vi "test_WFGenerate01DC.vi"() -> ()   [LabVIEW 2013]
panel:
  out "Waveform Out":waveform(dbl)={"t0"=timestamp(0 s since 1904-01-01), "dt"=5e-05, "Y"=array[10000 elements]}
  in  "Param 3":dbl=1000.0
  in  "Param 2":dbl=1000.0
  in  "Param 1":dbl=1000.0
  in  "Param 0":dbl=1000.0
  in  "Waveform Properties":T1={"Fs (Hz)"=20000.0, "Amplitude (V)"=5.0, "Ramp (s)"=0.02, "Duration (s)"=0.5} {"Ramp (s)" min=0.0; "Fs (Hz)" min=0.0}
  out "Waveform Graph":waveform(dbl)(graph)={"t0"=timestamp(0 s since 1904-01-01), "dt"=5e-05, "Y"=array[10000 elements]}
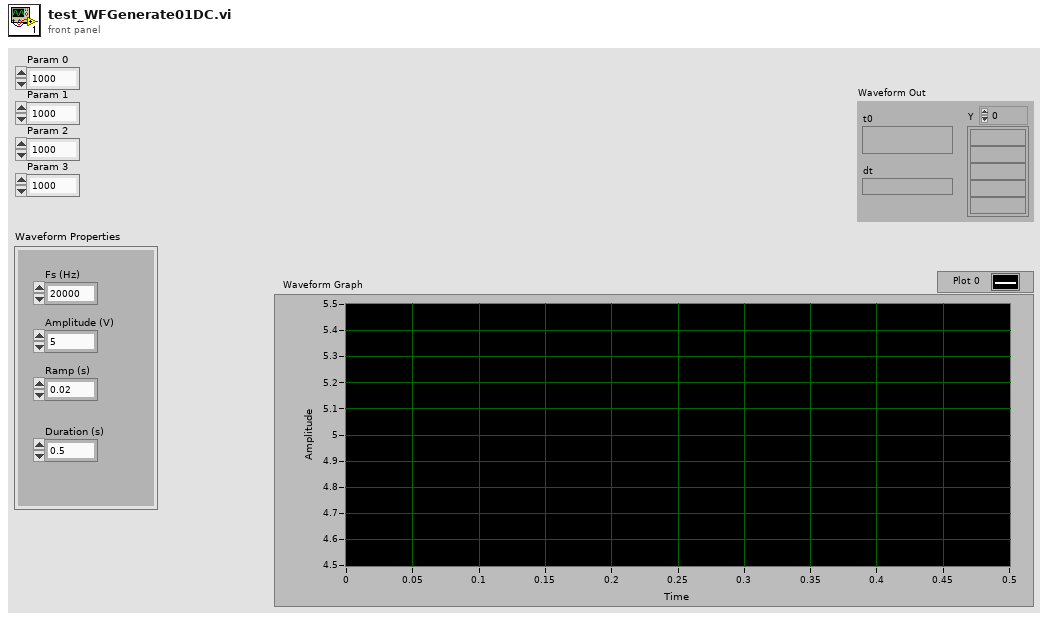
[diagram p1: front panel]
types:
  T1 = cluster{"Fs (Hz)":dbl, "Amplitude (V)":dbl, "Ramp (s)":dbl, "Duration (s)":dbl}
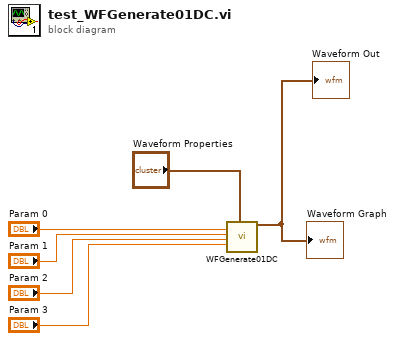
[diagram p0: block diagram]
diagram:
  n1 = call "WFGenerate01DC.vi"("Param 0"="Param 0", "Param 1"="Param 1", "Param 2"="Param 2", "Param 3"="Param 3", "Waveform Properties"="Waveform Properties") -> ("Waveform Out"=→"Waveform Graph" →"Waveform Out":waveform(dbl))  [unwired: 13 in, 1 out]
